vi "Calculate.vi"(8 "error in (no error)":errorcluster, 10 "Input String":string, 11 "Master Cluster":T1) -> (0 "error out":errorcluster, 1 "Data Entry Display":string, 2 "Result":dbl, 3 "Output M Cluster":T1)   [LabVIEW 2017]
uses:
  Controls/Master_Cluster.ctl
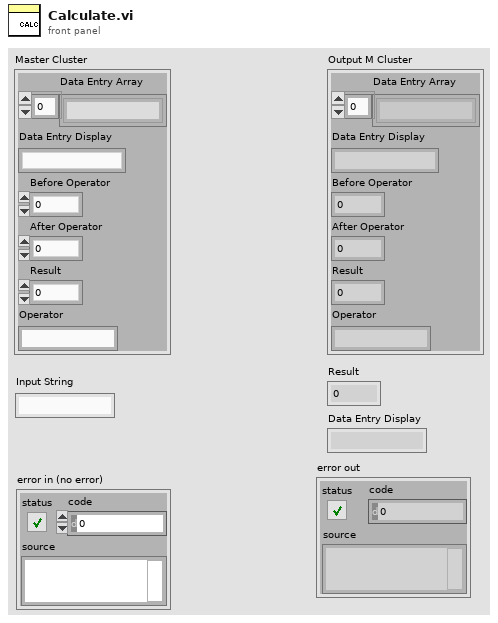
[diagram p1: front panel]
types:
  T1 = typedef "Master_Cluster.ctl" = cluster{"Data Entry Array":string[], "Data Entry Display":string, "Before Operator":dbl, "After Operator":dbl, "Result":dbl, "Operator":string}
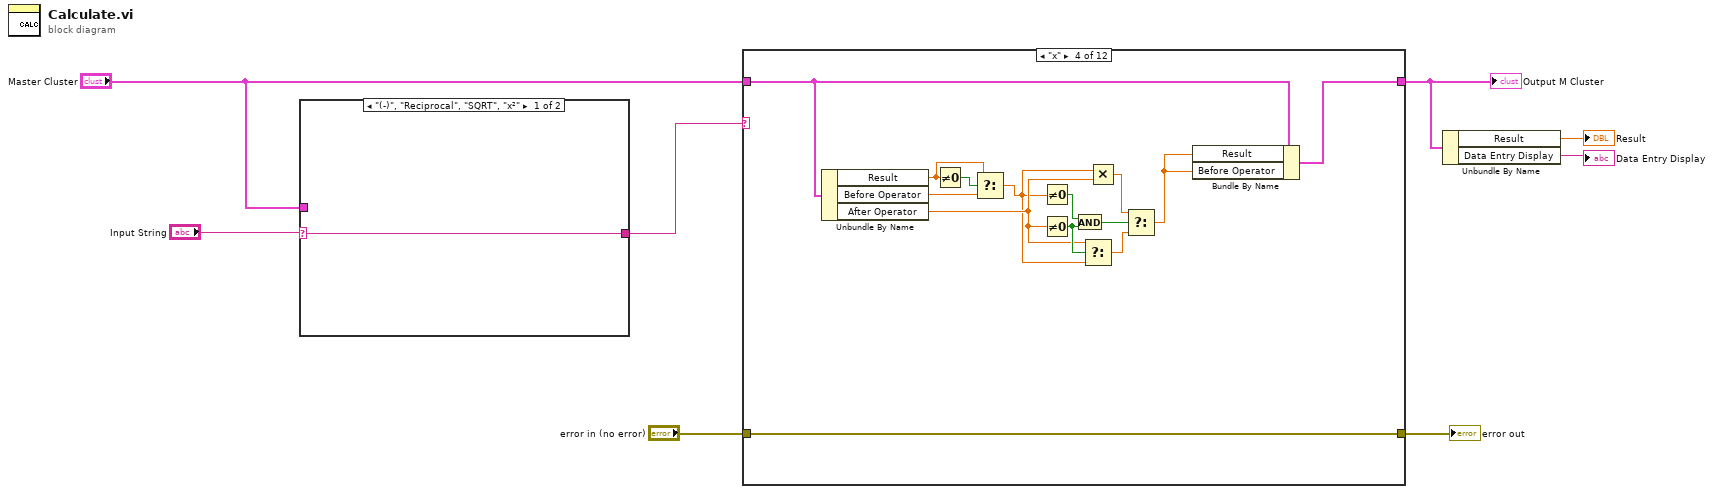
[diagram p0: block diagram]
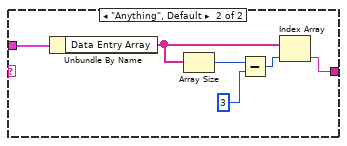
[diagram p2: hidden frame]
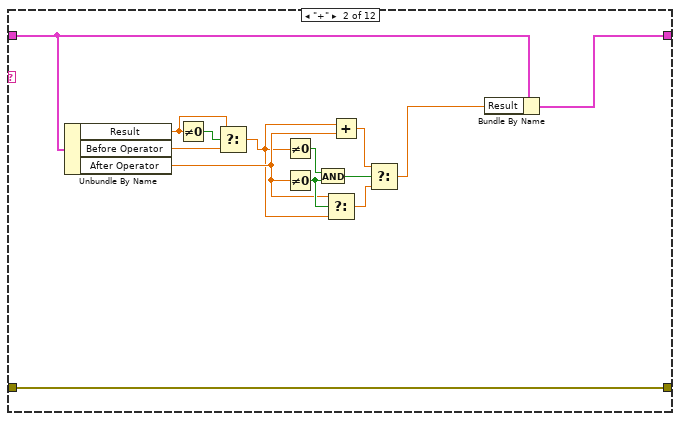
[diagram p4: hidden frame]
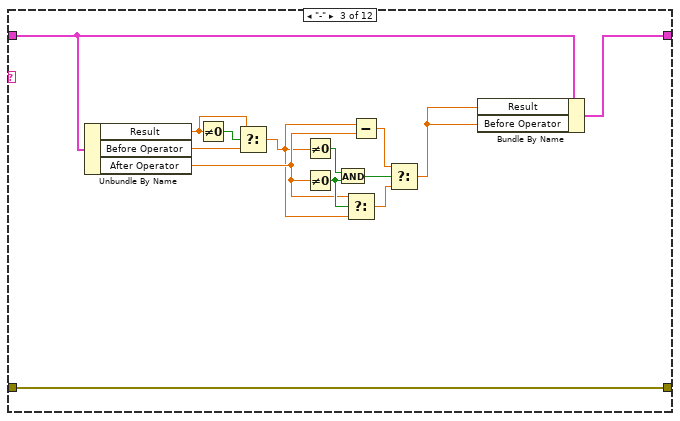
[diagram p5: hidden frame]
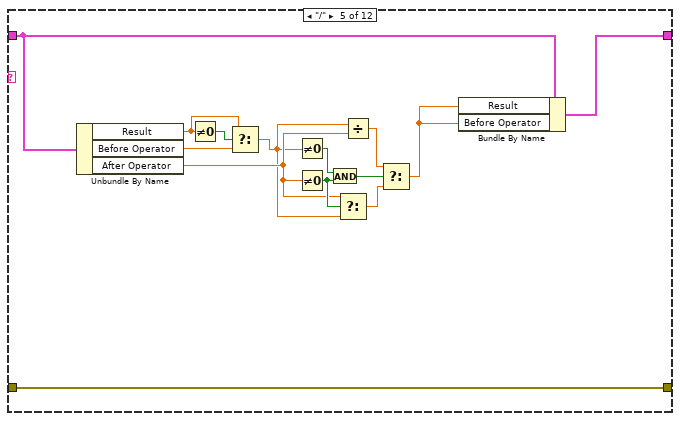
[diagram p6: hidden frame]
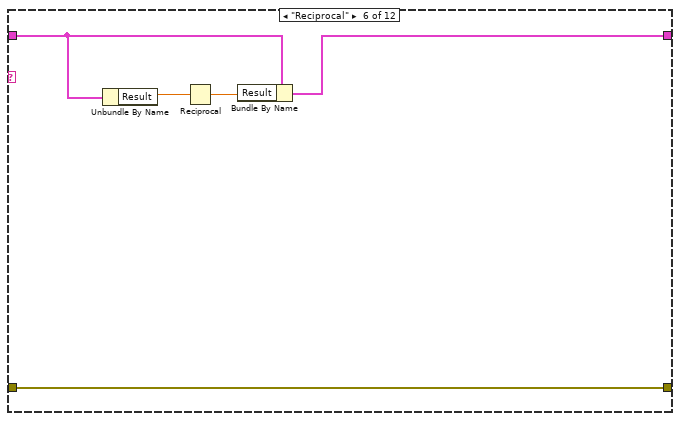
[diagram p7: hidden frame]
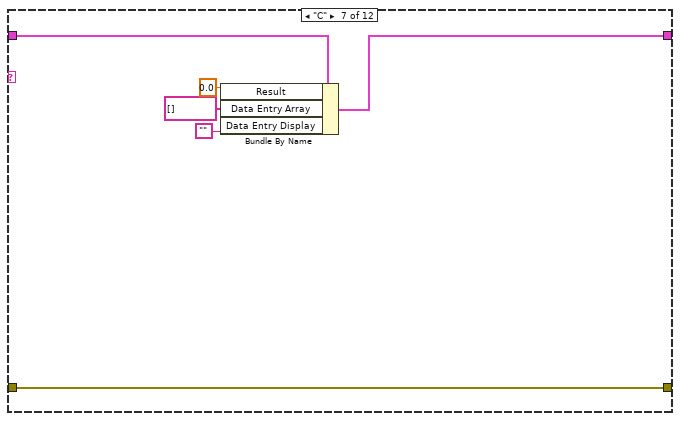
[diagram p8: hidden frame]
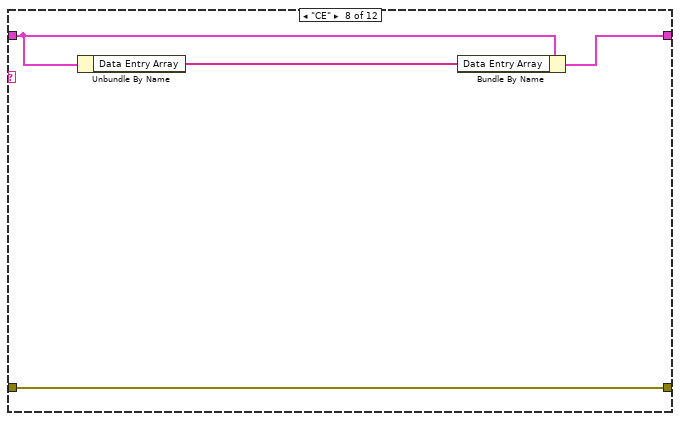
[diagram p9: hidden frame]
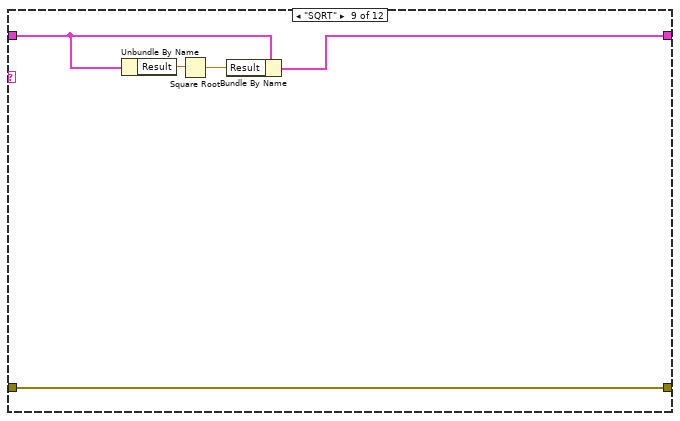
[diagram p10: hidden frame]
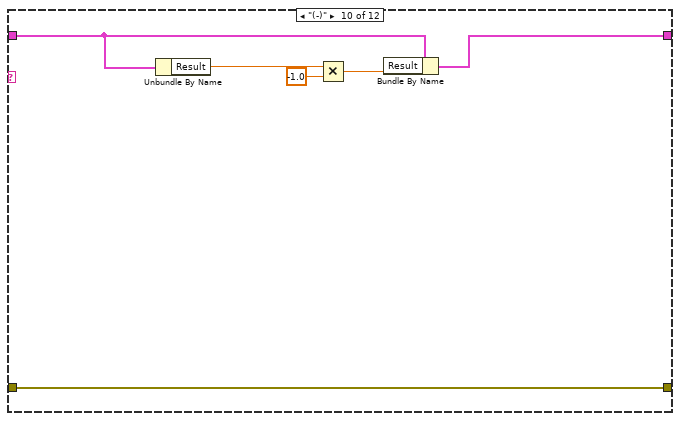
[diagram p11: hidden frame]
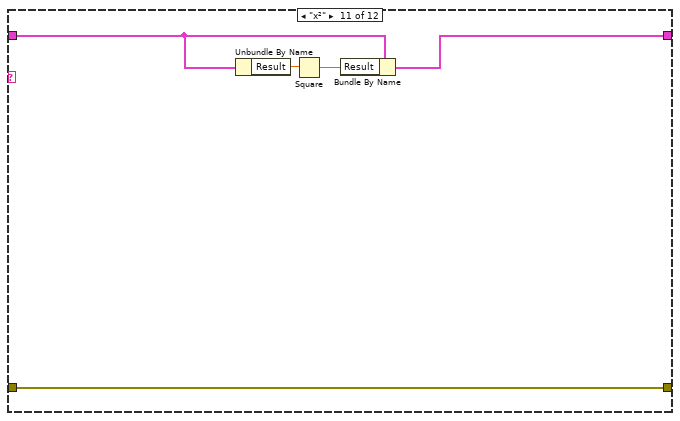
[diagram p12: hidden frame]
diagram:
  n1 = case shown="\"(-)\", \"Reciprocal\", \"SQRT\", \"x²\"" "Input String" {
    selector: "Input String" -> [w9 _]
    tunnel: "Master Cluster" -> [_ w11]
    tunnel: [w9 w10] -> w1
    frame "(-)", "Reciprocal", "SQRT", "x²" {
    }
    frame "Anything", Default {
      n2 = Unbundle By Name(w11) -> ("Data Entry Array"=w13:string[])
      n3 = Array Size(array=w13) -> (size(s)=w15:i32)
      n4 = Subtract(x=w15, y=3) -> (x-y=w14:i32)
      n5 = Index Array(array=w13, index=w14) -> (element=w10:string)
    }
  }
  n6 = case shown="\"x\"" w1 {
    tunnel: "Master Cluster" -> [w17 w26 w35 w49 w63 w78 w84 w88 w92 w98 w102 w105]
    tunnel: [w17 w25 w34 w48 w62 w77 w83 w87 w90 w97 w101 w105] -> w6
    tunnel: "error in (no error)" -> [w16 w19 w33 w47 w61 w74 w80 w86 w89 w94 w100 w106]
    tunnel: [w16 w19 w33 w47 w61 w74 w80 w86 w89 w94 w100 w106] -> w7
    frame "Invalid", Default {
    }
    frame "+" {
      n7 = Unbundle By Name(w26) -> ("Result"=w22:dbl, "Before Operator"=w21:dbl, "After Operator"=w24:dbl)
      n8 = Not Equal To 0?(x=w22) -> (x != 0?=w23:bool)
      n9 = Select(t=w22, s=w23, f=w21) -> (s? t:f=w20:dbl)
      n10 = Not Equal To 0?(x=w20) -> (x != 0?=w31:bool)
      n11 = Not Equal To 0?(x=w24) -> (x != 0?=w28:bool)
      n12 = And(x=w31, y=w28) -> (x .and. y?=w30:bool)
      n13 = Select(t=w24, s=w28, f=w20) -> (s? t:f=w27:dbl)
      n14 = Add(x=w20, y=w24) -> (x+y=w29:dbl)
      n15 = Select(t=w29, s=w30, f=w27) -> (s? t:f=w18:dbl)
      n16 = Bundle By Name(cluster=w26, "Result"=w18) -> (w25:T1)
    }
    frame "-" {
      n17 = Unbundle By Name(w35) -> ("Result"=w38:dbl, "Before Operator"=w37:dbl, "After Operator"=w40:dbl)
      n18 = Not Equal To 0?(x=w38) -> (x != 0?=w39:bool)
      n19 = Select(t=w38, s=w39, f=w37) -> (s? t:f=w36:dbl)
      n20 = Not Equal To 0?(x=w36) -> (x != 0?=w45:bool)
      n21 = Not Equal To 0?(x=w40) -> (x != 0?=w42:bool)
      n22 = And(x=w45, y=w42) -> (x .and. y?=w44:bool)
      n23 = Select(t=w40, s=w42, f=w36) -> (s? t:f=w41:dbl)
      n24 = Subtract(x=w36, y=w40) -> (x-y=w43:dbl)
      n25 = Select(t=w43, s=w44, f=w41) -> (s? t:f=w32:dbl)
      n26 = Bundle By Name(cluster=w35, "Result"=w32, "Before Operator"=w32) -> (w34:T1)
    }
    frame "x" {
      n27 = Unbundle By Name(w49) -> ("Result"=w52:dbl, "Before Operator"=w51:dbl, "After Operator"=w54:dbl)
      n28 = Not Equal To 0?(x=w52) -> (x != 0?=w53:bool)
      n29 = Select(t=w52, s=w53, f=w51) -> (s? t:f=w50:dbl)
      n30 = Not Equal To 0?(x=w50) -> (x != 0?=w59:bool)
      n31 = Not Equal To 0?(x=w54) -> (x != 0?=w56:bool)
      n32 = And(x=w59, y=w56) -> (x .and. y?=w58:bool)
      n33 = Select(t=w54, s=w56, f=w50) -> (s? t:f=w55:dbl)
      n34 = Multiply(x=w50, y=w54) -> (x*y=w57:dbl)
      n35 = Select(t=w57, s=w58, f=w55) -> (s? t:f=w46:dbl)
      n36 = Bundle By Name(cluster=w49, "Result"=w46, "Before Operator"=w46) -> (w48:T1)
    }
    frame "/" {
      n37 = Unbundle By Name(w63) -> ("Result"=w66:dbl, "Before Operator"=w65:dbl, "After Operator"=w68:dbl)
      n38 = Not Equal To 0?(x=w66) -> (x != 0?=w67:bool)
      n39 = Select(t=w66, s=w67, f=w65) -> (s? t:f=w64:dbl)
      n40 = Not Equal To 0?(x=w64) -> (x != 0?=w73:bool)
      n41 = Not Equal To 0?(x=w68) -> (x != 0?=w70:bool)
      n42 = And(x=w73, y=w70) -> (x .and. y?=w72:bool)
      n43 = Select(t=w68, s=w70, f=w64) -> (s? t:f=w69:dbl)
      n44 = Divide(x=w64, y=w68) -> (x/y=w71:dbl)
      n45 = Select(t=w71, s=w72, f=w69) -> (s? t:f=w60:dbl)
      n46 = Bundle By Name(cluster=w63, "Result"=w60, "Before Operator"=w60) -> (w62:T1)
    }
    frame "Reciprocal" {
      n47 = Unbundle By Name(w78) -> ("Result"=w76:dbl)
      n48 = Reciprocal(x=w76) -> (1/x=w75:dbl)
      n49 = Bundle By Name(cluster=w78, "Result"=w75) -> (w77:T1)
    }
    frame "C" {
      n50 = Bundle By Name(cluster=w84, "Result"=0.0, "Data Entry Array"=string[] [], "Data Entry Display"="") -> (w83:T1)
    }
    frame "CE" {
      n51 = Unbundle By Name(w88) -> ("Data Entry Array"=w85:string[])
      n52 = Bundle By Name(cluster=w88, "Data Entry Array"=w85) -> (w87:T1)
    }
    frame "SQRT" {
      n53 = Unbundle By Name(w92) -> ("Result"=w93:dbl)
      n54 = Square Root(x=w93) -> (sqrt(x)=w91:dbl)
      n55 = Bundle By Name(cluster=w92, "Result"=w91) -> (w90:T1)
    }
    frame "(-)" {
      n56 = Unbundle By Name(w98) -> ("Result"=w96:dbl)
      n57 = Multiply(x=w96, y=-1.0) -> (x*y=w99:dbl)
      n58 = Bundle By Name(cluster=w98, "Result"=w99) -> (w97:T1)
    }
    frame "x²" {
      n59 = Unbundle By Name(w102) -> ("Result"=w104:dbl)
      n60 = Square(x=w104) -> (x^2=w103:dbl)
      n61 = Bundle By Name(cluster=w102, "Result"=w103) -> (w101:T1)
    }
    frame "=" {
    }
  }
  "Output M Cluster" <- w6
  "error out" <- w7
  n62 = Unbundle By Name(w6) -> ("Result"=→"Result":dbl, "Data Entry Display"=→"Data Entry Display":string)
